vi "Uruchomienie_old.vi"() -> ()   [LabVIEW 2015]
uses:
  Typedefs/Analiza.ctl
  Typedefs/dane.ctl
  Typedefs/mqttinputs.ctl
  Libraries/MQTT.lvlibp
panel:
  in  "BtnStopPWM":bool
  out "Praca":bool
  out "DKG":bool
  in  "Cisnienie 2":T1 {"P" format="%#.1f"}
  in  "SKSVdial":T2 {"SV" format="%#.1f"; "SK" format="%#.1f"}
  in  "Start":bool
  out "Zapisane":bool
  in  "Do Bazy":bool
  out "Opis":string
  out "Tacho":dbl format="%#.0f"
  out "Moc Zamowiona":dbl
  out "Typ Palnika":string
  out "Typ Wymiennika":string
  out "SNW":string
  out "SNP":string
  out "cisnienieOK":bool
  in  "Cisnienie":bool
  in  "Analiza":T3 {"I" format="%#.0f"; "CO2" format="%#.1f"; "CO" format="%#.0f"; "O2" format="%#.1f"}
  out "SKSVOK":bool
  in  "SKSV":bool
  out "AnalizaMinKlientOK":bool
  out "AnalizaMaxKlientOK":bool
  out "AnalizaMinOK":bool
  out "AnalizaMaxOK":bool
  in  "AnalizaMinKlient":bool
  in  "AnalizaMaxKlient":bool
  in  "AnalizaMin":bool
  in  "AnalizaMax":bool
  in  "BtnMaxLufa":bool
  in  "BtnMin":bool
  in  "PWMMin":dbl=15.0
  in  "BtnMax Klient":bool
  in  "PWM Max Klient":dbl=90.0
  in  "Kas":bool
  out "Awaria":bool
  out "PWM":dbl
  in  "BtnMax":bool
  in  "PWM Max":dbl=100.0
  in  "BtnMin Klient":bool
  in  "PWMMinKlient":dbl=15.0
  in  "BtnStart":bool
  out "MOC":dbl format="%#_1g"
  in  "Uruchamia:":u16(ring) items=["------", "KAMIŃSKI JAKUB", "RADZIWON TOMASZ", "RADZIWON JAKUB", "RADZIWON MICHAŁ", "HARBANOWICZ FRANCISZEK", "JANUSZKIEWICZ JAKUB", "PIOTROWSKI DAMIAN", "WISZNIEWSKI JERZY", "BOHM ŁUKASZ", "KARPIŃSKI GRZEGORZ", "KAMIŃSKI JAKUB"]
  in  "Temat":u16(ring) items=["------"]
  in  "PWMStart":dbl=25.0
  in  "Nawiew_f":dbl=7.0
  in  "Nawiew":bool
  out "GAZ":bool
  in  "Zaplon":bool
  # "Hz"
  # "kW"
  # "21-24: 25%\npozostale 45%"
  # "%"
  # "%"
  # "Hz"
  # "%"
  # "%"
  # "%"
  # "%"
  # "Pa"
  # "mm"
  # "mm"
  # "Pmax 4%-5%\nPmin 3%-6.5%"
  # "%"
  # "%"
  # "ppm"
  # "<100ppm"
  # "uA"
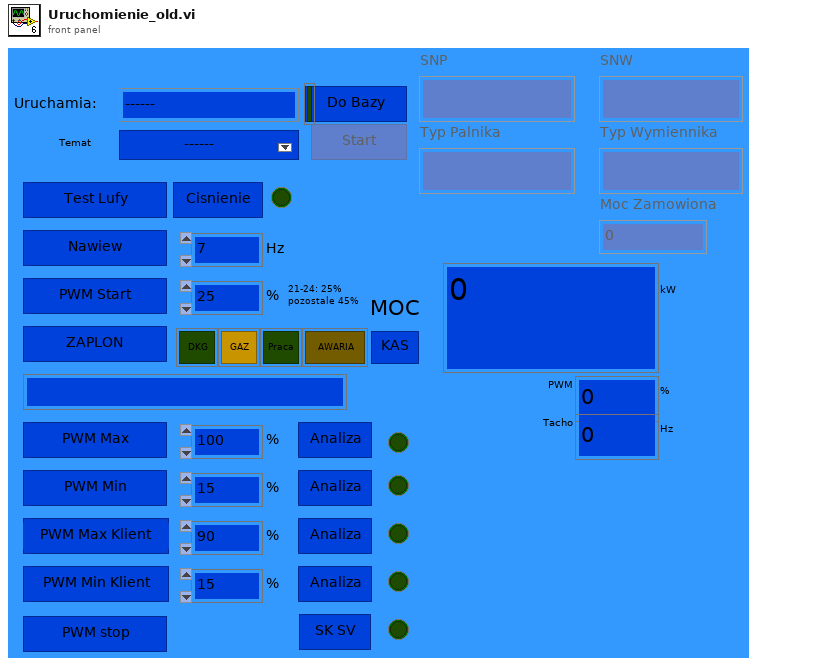
[diagram p1: front panel]
types:
  T1 = cluster{"P":dbl, "OK Button":bool, "Cancel Button":bool}
  T2 = cluster{"SK":dbl, "OK Button":bool, "Cancel Button":bool, "SV":dbl}
  T3 = typedef "Analiza.ctl" = cluster{"O2":dbl, "CO":dbl, "OK Button":bool, "Cancel Button":bool, "CO2":dbl, "I":dbl}
  T4 = typedef "MQTT.lvlibp/Broadcast Events--cluster.ctl" = cluster{"Module Did Init":refnum<user-event>, "Status Updated":refnum<user-event>, "Error Reported":refnum<user-event>, "Module Did Stop":refnum<user-event>, "Update Module Execution Status":refnum<user-event>, "Message":refnum<user-event>}
  T5 = enum8{"Enabled", "Disabled", "Disabled and Grayed Out"}
  T6 = enum32{"invalid app kind", "Development System", "Run Time System", "Student Edition", "Embedded LabVIEW", "Evaluation", "Custom"}
  T7 = typedef "dane.ctl" = cluster{"P":cluster{"max":dbl, "min":dbl, "klientmax":dbl, "klientmin":dbl}, "CO":cluster{"max":dbl, "min":dbl, "klientmax":dbl, "klientmin":dbl}, "CO2":cluster{"max":dbl, "min":dbl, "klientmax":dbl, "klientmin":dbl}, "O2":cluster{"max":dbl, "min":dbl, "klientmax":dbl, "klientmin":dbl}, "I":cluster{"max":dbl, "min":dbl, "klientmax":dbl, "klientmin":dbl}, "n":cluster{"max":dbl, "min":dbl, "klientmax":dbl, "klientmin":dbl}, "pwm":cluster{"klientmax":dbl, "klientmin":dbl}, "valve":cluster{"SK":dbl, "SV":dbl}, "pLufa100":dbl, "data":cluster{"Uruchomil":dbl, "Temat":string, "Podtemat":string, "Uwagi":string}}
  T8 = enum32{"Invalid", "Standard", "Closed", "Hidden", "Minimized", "Maximized"}
  T9 = typedef "mqttinputs.ctl" = cluster{"Power":dbl, "PWM":i32, "Tacho":i32, "Gaz":bool, "Awaria":bool, "dP":dbl, "Praca":bool, "DKG":bool}
  T10 = cluster{refnum<vi>[], "Core":cluster{"Current VI Reference":refnum<vi>, "Close Panel on Exit?":bool}, "controls":refnum<vi>[], "Kto-Lista":string[], "Kto-Lista-Num":i32[], "Kto":u8, "Tematy-Lista":string[], "TematyDane":string[][], "Temat":string, "Data":T7, "PWM":cluster{" start":i32, "min":i32, "max":i32, "moc":i32, "min klient":i32, "max klient":i32}, "CurrentPWM":i32, "broadcasts":variant, "Subscriptions":variant, "Inputs":T9, "Analiza":string}
  T11 = cluster{" start":i32, "min":i32, "max":i32, "moc":i32, "min klient":i32, "max klient":i32}
  T12 = cluster{"Current VI Reference":refnum<vi>, "Close Panel on Exit?":bool}
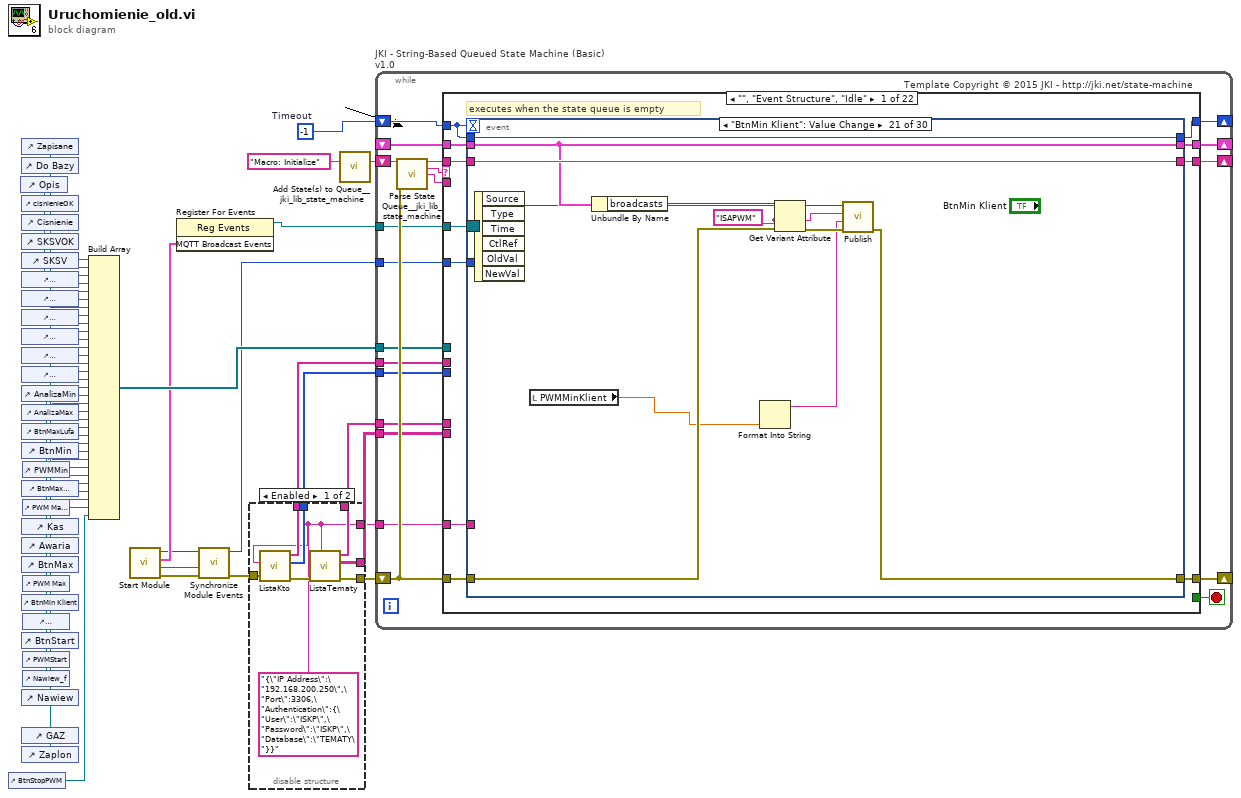
[diagram p0: block diagram]
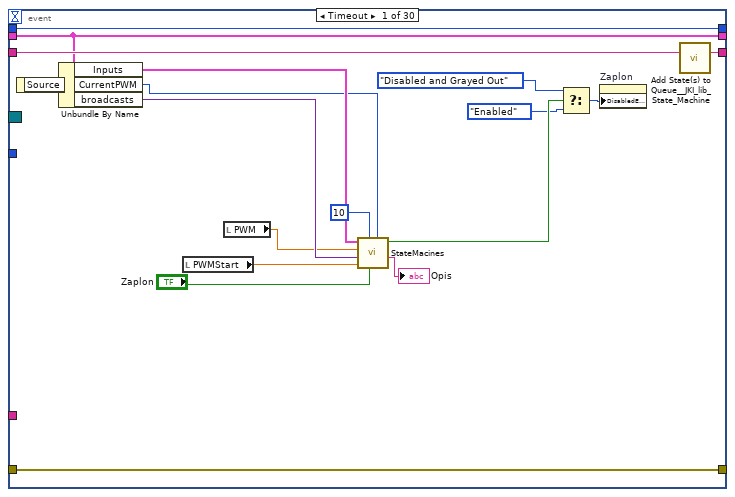
[diagram p3: hidden frame]
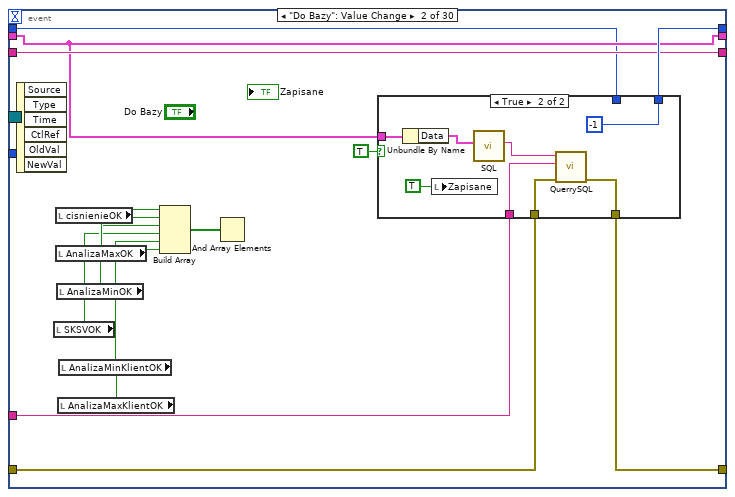
[diagram p4: hidden frame]
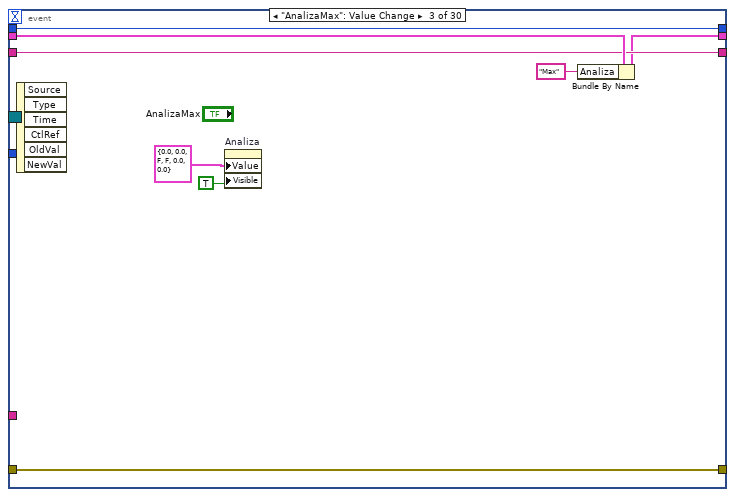
[diagram p6: hidden frame]
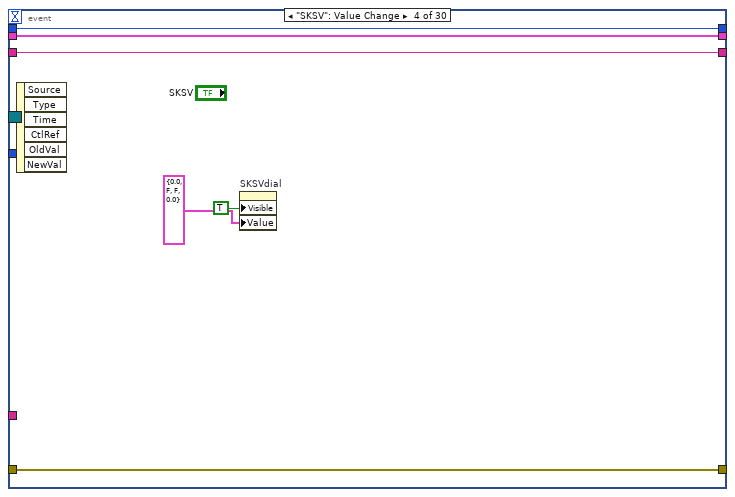
[diagram p7: hidden frame]
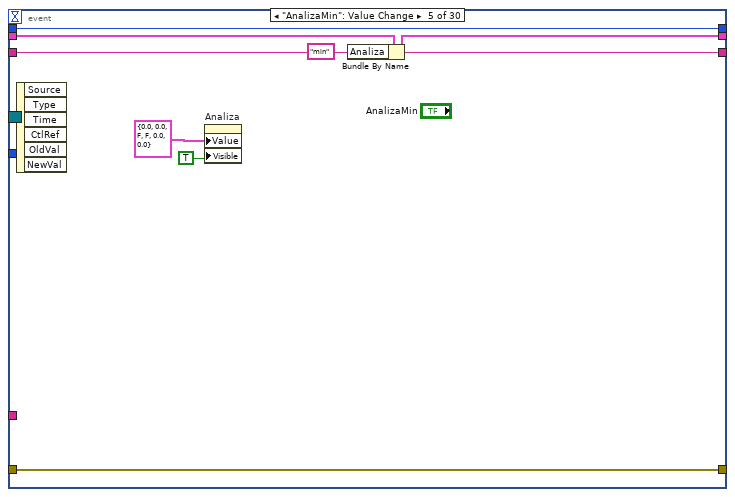
[diagram p8: hidden frame]
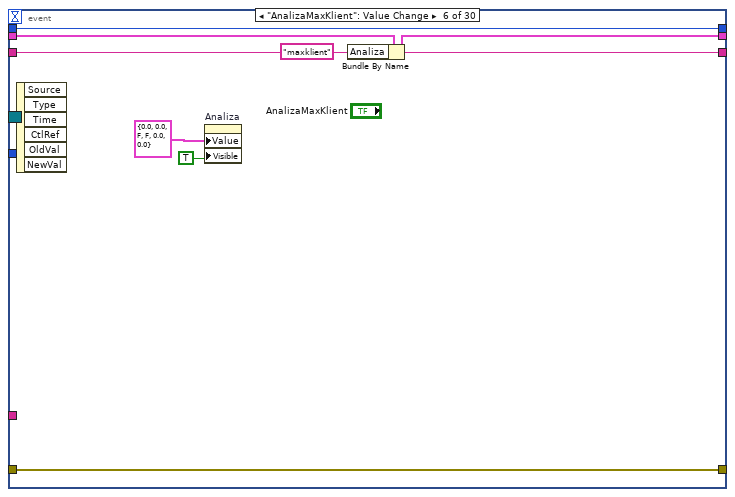
[diagram p9: hidden frame]
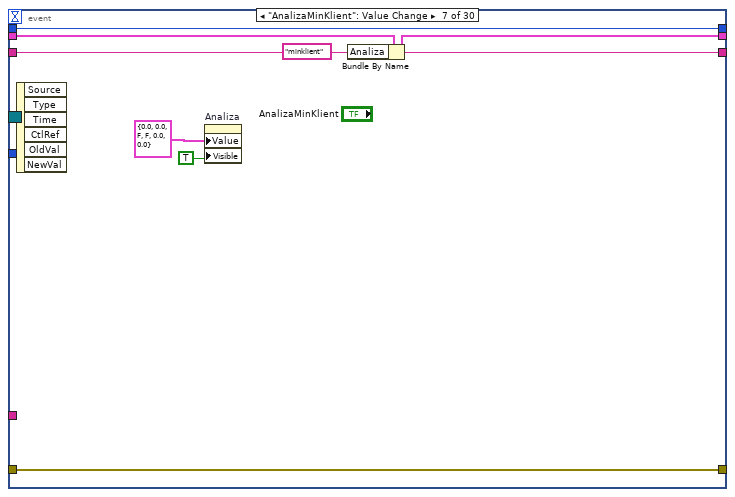
[diagram p10: hidden frame]
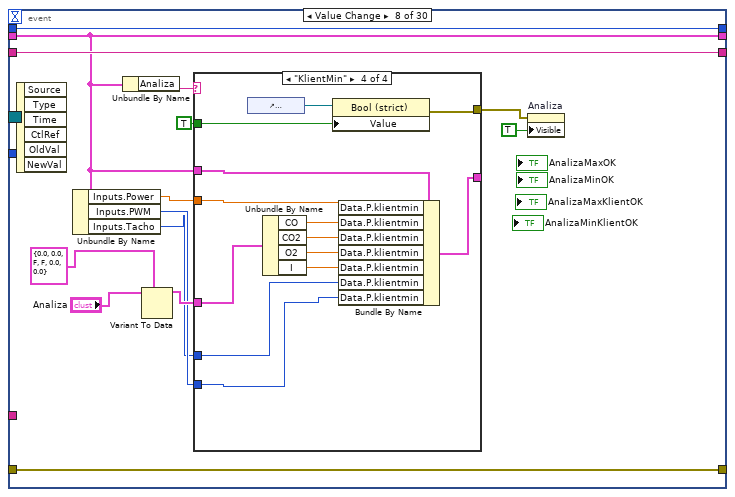
[diagram p11: hidden frame]
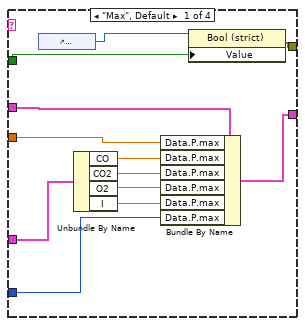
[diagram p12: hidden frame]
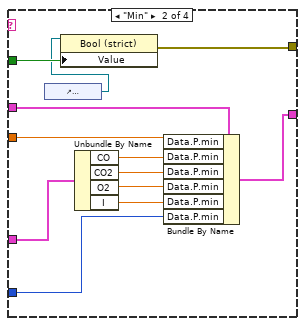
[diagram p13: hidden frame]
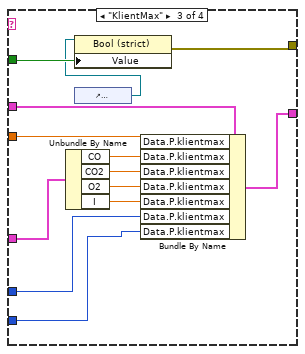
[diagram p14: hidden frame]
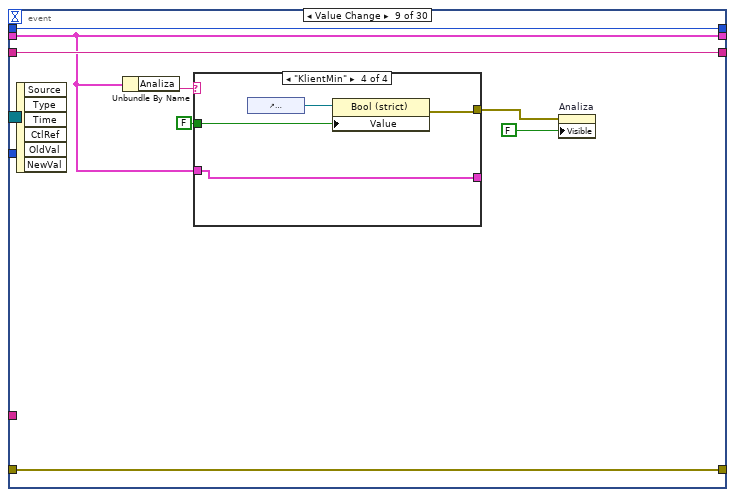
[diagram p15: hidden frame]
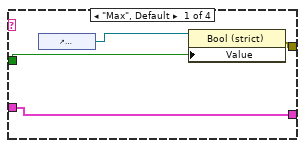
[diagram p16: hidden frame]
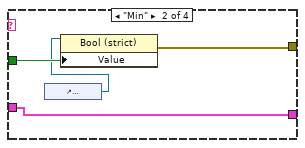
[diagram p17: hidden frame]
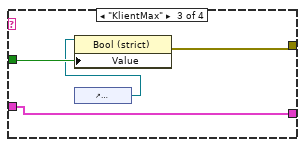
[diagram p18: hidden frame]
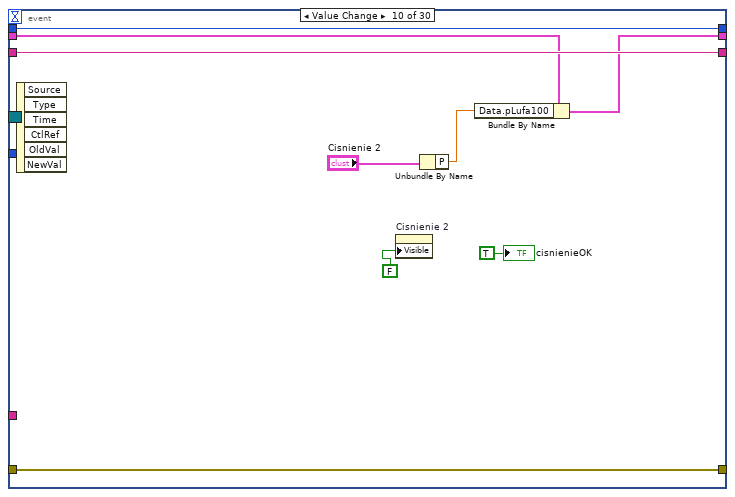
[diagram p19: hidden frame]
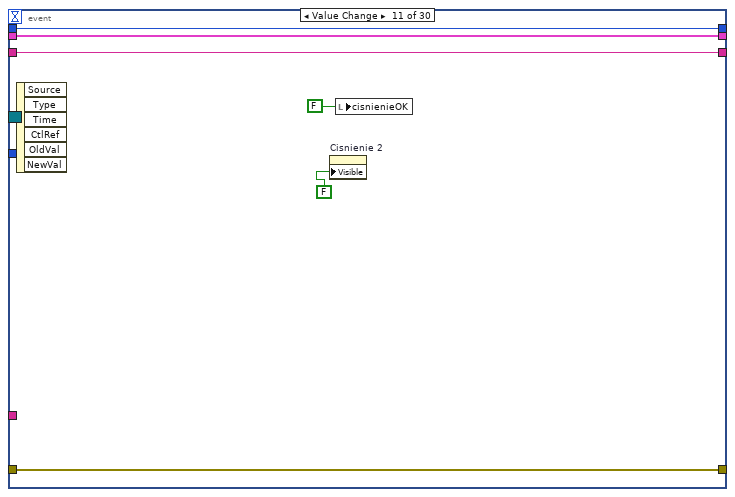
[diagram p20: hidden frame]
diagram:
  w3 = -1  # Timeout
  n1 = control-ref of="BtnStopPWM"() -> (w1:refnum<vi>)
  n2 = control-ref of="Opis"() -> (w48:refnum<vi>)
  n3 = control-ref of="Zapisane"() -> (w50:refnum<vi>)
  n4 = control-ref of="Do Bazy"() -> (w49:refnum<vi>)
  n5 = control-ref of="cisnienieOK"() -> (w47:refnum<vi>)
  n6 = control-ref of="Cisnienie"() -> (w46:refnum<vi>)
  n7 = control-ref of="SKSVOK"() -> (w45:refnum<vi>)
  n8 = control-ref of="SKSV"() -> (w44:refnum<vi>)
  n9 = control-ref of="AnalizaMinKlientOK"() -> (w43:refnum<vi>)
  n10 = control-ref of="AnalizaMaxKlientOK"() -> (w42:refnum<vi>)
  n11 = control-ref of="AnalizaMinOK"() -> (w41:refnum<vi>)
  n12 = control-ref of="AnalizaMaxOK"() -> (w40:refnum<vi>)
  n13 = control-ref of="AnalizaMinKlient"() -> (w39:refnum<vi>)
  n14 = control-ref of="AnalizaMaxKlient"() -> (w38:refnum<vi>)
  n15 = control-ref of="AnalizaMin"() -> (w37:refnum<vi>)
  n16 = control-ref of="AnalizaMax"() -> (w36:refnum<vi>)
  n17 = control-ref of="BtnMaxLufa"() -> (w35:refnum<vi>)
  n18 = control-ref of="BtnMin"() -> (w34:refnum<vi>)
  n19 = control-ref of="BtnMax Klient"() -> (w32:refnum<vi>)
  n20 = control-ref of="Kas"() -> (w30:refnum<vi>)
  n21 = control-ref of="Awaria"() -> (w29:refnum<vi>)
  n22 = control-ref of="BtnMax"() -> (w28:refnum<vi>)
  n23 = control-ref of="BtnMin Klient"() -> (w26:refnum<vi>)
  n24 = control-ref of="BtnStart"() -> (w24:refnum<vi>)
  n25 = control-ref of="Nawiew"() -> (w21:refnum<vi>)
  n26 = control-ref of="GAZ"() -> (w20:refnum<vi>)
  n27 = control-ref of="Zaplon"() -> (w19:refnum<vi>)
  n28 = control-ref of="PWMMin"() -> (w33:refnum<vi>)
  n29 = control-ref of="PWM Max Klient"() -> (w31:refnum<vi>)
  n30 = control-ref of="PWM Max"() -> (w27:refnum<vi>)
  n31 = control-ref of="PWMMinKlient"() -> (w25:refnum<vi>)
  n32 = control-ref of="PWMStart"() -> (w23:refnum<vi>)
  n33 = control-ref of="Nawiew_f"() -> (w22:refnum<vi>)
  n34 = Build Array(w50, w49, w48, w47, w46, w45, w44, w43, w42, w41, w40, w39, w38, w37, w36, w35, w34, w33, w32, w31, w30, w29, w28, w27, w26, w25, w24, w23, w22, w21, w20, w19, w1) -> (w11:refnum<vi>[])
  n35 = call "Start Module.vi"() -> ("error out"=w6:errorcluster, "Wait for Event Sync?"=w7:bool, "MQTT Broadcast Events"=w10:T4, "Module ID"=w9:i32)  [unwired: 8 in]
  n36 = register-events(w10) -> (reference out=w4:refnum<event-registration>)  [unwired: 2 in, 1 out]
  n37 = call "Synchronize Module Events.vi"("error in (no error)"=w6, "Wait for Event Sync?"=w7, "Module ID"=w9) -> ("error out"=w5:errorcluster, "Module ID (dup)"=w8:i32)  [unwired: 7 in]
  n38 = disable-structure shown="Enabled" {
    disable-tunnel: [w58 w59] -> w16
    disable-tunnel: [w56 _] -> w15
    disable-tunnel: [w55 _] -> w14
    disable-tunnel: [w54 _] -> w13
    disable-tunnel: [w53 _] -> w12
    disable-tunnel: w5 -> [w52 w59]
    disable-tunnel: [w51 _] -> w2
    frame Enabled {
      w51 = "{\"IP Address\":\"192.168.200.250\",\"Port\":3306,\"Authentication\":{\"User\":\"ISKP\",\"Password\":\"ISKP\",\"Database\":\"TEMATY\"}}" ("JSON string")
      n39 = call "ListaKto.vi"("error in (no error)"=w52, "Jsonconfig"=w51) -> ("error out"=w57:errorcluster, "Array"=w55:i32[], "Array 2"=w56:string[])  [unwired: 7 in]
      n40 = call "ListaTematy.vi"("Jsonconfig"=w51, "error in (no error)"=w57) -> ("error out"=w58:errorcluster, "data"=w53:string[][], "Array"=w54:string[])  [unwired: 7 in]
    }
    frame Disabled {
    }
  }
  n41 = call <vilib>:"Add State(s) to Queue__jki_lib_state_machine.vi"("State(s) in (\"\")"="Macro: Initialize") -> ("States Out"=w18:string)  [unwired: 14 in]
  n42 = while "JKI - String-Based Queued State Machine (Basic) v1.0" {
    shift-right: [w72] -> _
    shift-left: _ -> [w71]
    shift-right: [w75] -> _
    shift-left: w16 -> [w70]
    shift-right: [w74] -> _
    shift-left: w18 -> [w76]
    tunnel: w15 -> [w69]
    tunnel: w14 -> [w68]
    tunnel: w13 -> [w67]
    tunnel: w12 -> [w66]
    tunnel: w11 -> [w65]
    tunnel: w8 -> [w64]
    tunnel: w4 -> [w63]
    shift-right: [w61] -> _
    shift-left: w3 -> [w62]
    tunnel: w2 -> [w60]
    stop <- w73 stop-if-true
    # "Template Copyright © 2015 JKI - http://jki.net/state-machine"
    n43 = call <vilib>:"Parse State Queue__jki_lib_state_machine.vi"("State Queue"=w76, "Error In (no error)"=w70) -> ("Remaining States"=w78:string, "Current State"=w79:string, "Arguments"=w77:string)  [unwired: 11 in]
    n44 = case shown="\"\", \"Event Structure\", \"Idle\"" w79 {
      selector: w79 -> [_ _ w543 _ _ _ _ _ _ _ _ _ _ _ _ _ _ _ _ _ _ _]
      tunnel: w78 -> [w90 w541 w547 w567 w574 w585 w590 w619 w626 w631 w642 w647 w654 w670 w679 w691 w718 w724 w735 w740 w745 w750]
      tunnel: w77 -> [_ _ _ _ _ _ _ _ _ _ _ _ _ w655 w674 w685 _ _ _ _ _ _]
      tunnel: w71 -> [w88 w538 w545 w558 w571 w583 w587 _ w621 w628 w636 w644 w650 w666 w677 w687 w715 w721 w732 w737 w742 w747]
      tunnel: [w87 w539 w549 w564 errorcluster {"status"=FALSE, "code"=0, "source"=""} ("error out") w576 w588 w616 w622 w629 w638 w645 w652 w668 w675 w688 w716 w722 w733 w738 w743 w748] -> w75
      tunnel: w70 -> [w86 w539 w548 w564 w570 w577 w588 w616 w623 w629 w639 w645 w652 w668 w676 w689 w716 w722 w733 w738 w743 w748]
      tunnel: [w89 w540 w546 w566 w573 w584 w589 w618 w625 w630 w641 w646 w653 w669 w678 w690 w717 w723 w734 w739 w744 w749] -> w74
      tunnel: [_ _ _ _ _ TRUE _ _ _ _ _ _ _ _ _ _ _ _ _ _ _ _] -> w73
      tunnel: [w85 w538 w545 w565 w571 w583 w587 w617 w621 w628 w635 w644 w650 w666 w677 w687 w715 w721 w732 w737 w742 w747] -> w72
      tunnel: w62 -> [w82 w537 w542 w555 w568 w575 w586 w592 w620 w627 w632 w643 w651 w656 w673 w684 w714 w719 w725 w736 w741 w746]
      tunnel: w69 -> [_ _ _ _ _ _ _ w603 _ _ _ _ _ _ _ _ _ _ _ _ _ _]
      tunnel: w68 -> [_ _ _ _ _ _ _ w602 _ _ _ _ _ _ _ _ _ _ _ _ _ _]
      tunnel: w67 -> [_ _ _ _ _ _ _ w601 _ _ _ _ _ _ _ _ _ _ _ _ _ _]
      tunnel: w66 -> [_ _ _ _ _ _ _ w600 _ _ _ _ _ _ _ _ _ _ _ _ _ _]
      tunnel: w65 -> [_ _ _ w554 _ _ _ w598 _ _ _ _ _ _ _ _ _ _ _ _ _ _]
      tunnel: w64 -> [w84 _ _ _ _ w578 _ _ _ _ w640 _ _ _ _ _ _ _ _ _ _ _]
      tunnel: w63 -> [w83 _ _ _ _ w581 _ _ _ _ _ _ _ _ _ _ _ _ _ _ _ _]
      tunnel: [w81 w537 w542 w555 w568 w575 w586 w592 w620 w627 w632 w643 w651 w656 w673 w684 w714 w719 w725 w736 w741 w746] -> w61
      tunnel: w60 -> [w80 _ _ _ _ _ _ _ _ _ _ _ _ _ _ _ _ _ _ _ _ _]
      frame "", "Event Structure", "Idle" {
        # "executes when the state queue is empty"
        n45 = event shown="[20] \"BtnMin Klient\": Value Change" {
          selector: w83 -> [_ _ _ _ _ _ _ _ _ _ _ _ _ _ _ _ _ _ _ _ _ _ _ _ _ _ _ _ _ _]
          dyn-events: _ -> [_ _ _ _ _ _ _ _ _ _ _ _ _ _ _ _ _ _ _ _ _ _ _ _ _ _ _ _ _ _]
          timeout: w82 -> [_ _ _ _ _ _ _ _ _ _ _ _ _ _ _ _ _ _ _ _ _ _ _ _ _ _ _ _ _ _]
          tunnel: w90 -> [w107 w121 w137 w146 w154 w162 w170 w184 w242 w267 w273 w283 w289 w295 w315 w329 w338 w363 w375 w386 w398 w410 w422 w434 w454 w464 w498 w504 w526 w536]
          tunnel: [w106 w121 w137 w146 w154 w162 w170 w184 w242 w267 w273 w283 w289 w295 w315 w329 w338 w363 w375 w386 w398 w410 w422 w434 w454 w464 w498 w505 w526 w535] -> w89
          tunnel: w88 -> [w100 w120 w138 w144 w152 w160 w168 w174 w237 w263 w271 w277 w287 w293 w313 w327 w336 w361 w373 w384 w396 w408 w420 w432 w452 w457 w496 w506 w524 w533]
          tunnel: [w105 w117 w139 w145 w153 w161 w169 w183 w241 w266 w272 w282 w288 w294 w301 w321 w333 w358 w370 w381 w393 w405 w417 w429 w436 w459 w494 w502 w509 w534] -> w87
          tunnel: w86 -> [w105 w118 w139 w145 w153 w161 w169 w183 w241 w266 w272 w282 w288 w294 w302 w320 w332 w357 w369 w380 w392 w404 w416 w428 w447 w459 w494 w502 w509 w534]
          tunnel: [w100 w120 w136 w144 w148 w156 w164 w174 w237 w262 w271 w276 w287 w293 w313 w327 w336 w361 w373 w384 w396 w408 w420 w432 w452 w456 w495 w506 w525 w533] -> w85
          tunnel: w84 -> [_ _ _ _ _ _ _ _ _ _ _ _ _ _ w305 w323 w334 w359 w371 w382 w394 w406 w418 w430 w438 _ _ _ _ _]
          tunnel: w82 -> [w97 w108 w140 w143 w151 w159 w167 w182 w240 w265 w270 w281 w286 w292 w314 w328 w337 w362 w374 w385 w397 w409 w421 w433 w453 w455 w493 _ w507 w530]
          tunnel: [w97 w122 w140 w143 w151 w159 w167 w182 w240 w265 w270 w281 w286 w292 w314 w328 w337 w362 w374 w385 w397 w409 w421 w433 w453 w455 w493 500 ("Timeout") w507 w530] -> w81
          tunnel: w80 -> [_ w119 _ _ _ _ _ _ _ _ _ _ _ _ _ _ _ _ _ _ _ _ _ _ _ _ _ _ _ _]
          event Timeout {
            n46 = event-data() -> ()  [unwired: 1 in, 1 out]
            n47 = Unbundle By Name(w100) -> ("Inputs"=w99:T9, "CurrentPWM"=w91:i32, "broadcasts"=w98:variant)
            n48 = local read "PWMStart"() -> (w96:dbl)
            n49 = local read "PWM"() -> (w93:dbl)
            n50 = call "StateMacines.vi"("PWM Demand"=w91, "Operate"="Zaplon", "Purge Time"=10, "PWMStart"=w96, "broadcasts"=w98, "CurrentPWM"=w93, "Inputs"=w99) -> ("Opis"=→"Opis":string, "DisableStartBtn"=w104:bool)  [unwired: 1 in, 2 out]
            n51 = Select(t=T5."Disabled and Grayed Out" ("Disabled"), s=w104, f=T5."Enabled" ("Disabled")) -> (s? t:f=w101:T5)
            n52 = property on="Zaplon" class="Bool (strict)"("DisabledEnum"=w101) -> ()  [unwired: 2 in, 2 out]
            n53 = call <vilib>:"Add State(s) to Queue__JKI_lib_State_Machine.vi"("State(s) in (\"\")"=w107) -> ("States Out"=w106:string)  [unwired: 14 in]
          }
          event "Do Bazy": Value Change {
            n54 = event-data() -> ()  [unwired: 1 in, 6 out]
            n55 = local read "SKSVOK"() -> (w113:bool)
            n56 = local read "cisnienieOK"() -> (w116:bool)
            n57 = local read "AnalizaMaxOK"() -> (w115:bool)
            n58 = local read "AnalizaMinOK"() -> (w114:bool)
            n59 = local read "AnalizaMaxKlientOK"() -> (w111:bool)
            n60 = local read "AnalizaMinKlientOK"() -> (w112:bool)
            n61 = Build Array(w116, w115, w114, w113, w112, w111) -> (w110:bool[])
            n62 = And Array Elements(Boolean array=w110) -> ()  [unwired: 1 out]
            n63 = case shown="True" TRUE {
              tunnel: [w123 -1 ("Timeout")] -> w122
              tunnel: w120 -> [_ w131]
              tunnel: w119 -> [_ w128]
              tunnel: w118 -> [w124 w127]
              tunnel: [w124 w126] -> w117
              tunnel: w108 -> [w123 _]
              frame False {
              }
              frame True {
                n64 = Unbundle By Name(w131) -> ("Data"=w130:T7)
                n65 = local write "Zapisane"(TRUE ("Zapisane")) -> ()
                n66 = call "SQL.vi"("Data"=w130) -> ("SQL querry"=w129:string)  [unwired: 9 in, 1 out]
                n67 = call "QuerrySQL.vi"("error in (no error)"=w127, "Jsonconfig"=w128, "String"=w129) -> ("error out"=w126:errorcluster)  [unwired: 7 in, 1 out]
              }
            }
          }
          event "AnalizaMax": Value Change {
            n68 = event-data() -> ()  [unwired: 1 in, 6 out]
            n69 = property on="Analiza" class="Clust"("Value"=T3 {"O2"=0.0, "CO"=0.0, "OK Button"=FALSE, "Cancel Button"=FALSE, "CO2"=0.0, "I"=0.0} ("Analiza"), "Visible"=TRUE) -> ()  [unwired: 2 in, 2 out]
            n70 = Bundle By Name(cluster=w138, "Analiza"="Max") -> (w136:T10)
          }
          event "SKSV": Value Change {
            n71 = event-data() -> ()  [unwired: 1 in, 6 out]
            n72 = property on="SKSVdial" class="Clust"("Visible"=TRUE, "Value"=T2 {"SK"=0.0, "OK Button"=FALSE, "Cancel Button"=FALSE, "SV"=0.0} ("SKSV")) -> ()  [unwired: 2 in, 2 out]
          }
          event "AnalizaMin": Value Change {
            n73 = event-data() -> ()  [unwired: 1 in, 6 out]
            n74 = property on="Analiza" class="Clust"("Value"=T3 {"O2"=0.0, "CO"=0.0, "OK Button"=FALSE, "Cancel Button"=FALSE, "CO2"=0.0, "I"=0.0} ("Analiza"), "Visible"=TRUE) -> ()  [unwired: 2 in, 2 out]
            n75 = Bundle By Name(cluster=w152, "Analiza"="min") -> (w148:T10)
          }
          event "AnalizaMaxKlient": Value Change {
            n76 = event-data() -> ()  [unwired: 1 in, 6 out]
            n77 = property on="Analiza" class="Clust"("Value"=T3 {"O2"=0.0, "CO"=0.0, "OK Button"=FALSE, "Cancel Button"=FALSE, "CO2"=0.0, "I"=0.0} ("Analiza"), "Visible"=TRUE) -> ()  [unwired: 2 in, 2 out]
            n78 = Bundle By Name(cluster=w160, "Analiza"="maxklient") -> (w156:T10)
          }
          event "AnalizaMinKlient": Value Change {
            n79 = event-data() -> ()  [unwired: 1 in, 6 out]
            n80 = property on="Analiza" class="Clust"("Value"=T3 {"O2"=0.0, "CO"=0.0, "OK Button"=FALSE, "Cancel Button"=FALSE, "CO2"=0.0, "I"=0.0} ("Analiza"), "Visible"=TRUE) -> ()  [unwired: 2 in, 2 out]
            n81 = Bundle By Name(cluster=w168, "Analiza"="minklient") -> (w164:T10)
          }
          event Value Change {
            n82 = event-data() -> ()  [unwired: 1 in, 6 out]
            n83 = Unbundle By Name(w174) -> ("Inputs.Power"=w173:dbl, "Inputs.PWM"=w172:i32, "Inputs.Tacho"=w171:i32)
            n84 = Unbundle By Name(w174) -> ("Analiza"=w178:string)
            n85 = Variant To Data(type=T3 {"O2"=0.0, "CO"=0.0, "OK Button"=FALSE, "Cancel Button"=FALSE, "CO2"=0.0, "I"=0.0} ("Analiza"), Variant="Analiza") -> (data=w180:T3)  [unwired: 1 in, 1 out]
            n86 = case shown="\"KlientMin\"" w178 {
              tunnel: TRUE ("AnalizaMinOK") -> [w196 w208 w221 w234]
              tunnel: [w195 w207 w220 w233] -> w177
              tunnel: [w190 w202 w218 w227] -> _
              tunnel: w174 -> [w189 w201 w219 w228]
              tunnel: w180 -> [w188 w199 w217 w225]
              tunnel: w173 -> [w187 w200 w212 w226]
              tunnel: w171 -> [w186 w198 w211 w224]
              tunnel: w172 -> [_ _ w210 w223]
              frame "Max", Default {
                n87 = control-ref of="AnalizaMaxOK"() -> (w185:refnum<vi>)
                n88 = Unbundle By Name(w188) -> ("CO"=w194:dbl, "CO2"=w193:dbl, "O2"=w192:dbl, "I"=w191:dbl)
                n89 = Bundle By Name(cluster=w189, "Data.P.max"=w187, "Data.P.max"=w194, "Data.P.max"=w193, "Data.P.max"=w192, "Data.P.max"=w191, "Data.P.max"=w186) -> (w190:T10)
                n90 = property on="Property Node" class="Bool (strict)"(reference=w185, "Value"=w196) -> (error out=w195:errorcluster)  [unwired: 1 in, 1 out]
              }
              frame "Min" {
                n91 = control-ref of="AnalizaMinOK"() -> (w197:refnum<vi>)
                n92 = property on="Property Node" class="Bool (strict)"(reference=w197, "Value"=w208) -> (error out=w207:errorcluster)  [unwired: 1 in, 1 out]
                n93 = Unbundle By Name(w199) -> ("CO"=w206:dbl, "CO2"=w205:dbl, "O2"=w204:dbl, "I"=w203:dbl)
                n94 = Bundle By Name(cluster=w201, "Data.P.min"=w200, "Data.P.min"=w206, "Data.P.min"=w205, "Data.P.min"=w204, "Data.P.min"=w203, "Data.P.min"=w198) -> (w202:T10)
              }
              frame "KlientMax" {
                n95 = Unbundle By Name(w217) -> ("CO"=w213:dbl, "CO2"=w214:dbl, "O2"=w215:dbl, "I"=w216:dbl)
                n96 = control-ref of="AnalizaMaxKlientOK"() -> (w209:refnum<vi>)
                n97 = property on="Property Node" class="Bool (strict)"(reference=w209, "Value"=w221) -> (error out=w220:errorcluster)  [unwired: 1 in, 1 out]
                n98 = Bundle By Name(cluster=w219, "Data.P.klientmax"=w212, "Data.P.klientmax"=w213, "Data.P.klientmax"=w214, "Data.P.klientmax"=w215, "Data.P.klientmax"=w216, "Data.P.klientmax"=w211, "Data.P.klientmax"=w210) -> (w218:T10)
              }
              frame "KlientMin" {
                n99 = control-ref of="AnalizaMinKlientOK"() -> (w222:refnum<vi>)
                n100 = Unbundle By Name(w225) -> ("CO"=w232:dbl, "CO2"=w231:dbl, "O2"=w230:dbl, "I"=w229:dbl)
                n101 = property on="Property Node" class="Bool (strict)"(reference=w222, "Value"=w234) -> (error out=w233:errorcluster)  [unwired: 1 in, 1 out]
                n102 = Bundle By Name(cluster=w228, "Data.P.klientmin"=w226, "Data.P.klientmin"=w232, "Data.P.klientmin"=w231, "Data.P.klientmin"=w230, "Data.P.klientmin"=w229, "Data.P.klientmin"=w224, "Data.P.klientmin"=w223) -> (w227:T10)
              }
            }
            n103 = property on="Analiza" class="Clust"(error in=w177, "Visible"=TRUE) -> ()  [unwired: 1 in, 2 out]
          }
          event Value Change {
            n104 = event-data() -> ()  [unwired: 1 in, 6 out]
            n105 = Unbundle By Name(w237) -> ("Analiza"=w239:string)
            n106 = case shown="\"KlientMin\"" w239 {
              tunnel: FALSE ("AnalizaMinOK") -> [w246 w250 w254 w258]
              tunnel: [w245 w249 w253 w257] -> w236
              tunnel: [w244 w248 w252 w256] -> _
              tunnel: w237 -> [w244 w248 w252 w256]
              frame "Max", Default {
                n107 = control-ref of="AnalizaMaxOK"() -> (w243:refnum<vi>)
                n108 = property on="Property Node" class="Bool (strict)"(reference=w243, "Value"=w246) -> (error out=w245:errorcluster)  [unwired: 1 in, 1 out]
              }
              frame "Min" {
                n109 = control-ref of="AnalizaMinOK"() -> (w247:refnum<vi>)
                n110 = property on="Property Node" class="Bool (strict)"(reference=w247, "Value"=w250) -> (error out=w249:errorcluster)  [unwired: 1 in, 1 out]
              }
              frame "KlientMax" {
                n111 = control-ref of="AnalizaMaxKlientOK"() -> (w251:refnum<vi>)
                n112 = property on="Property Node" class="Bool (strict)"(reference=w251, "Value"=w254) -> (error out=w253:errorcluster)  [unwired: 1 in, 1 out]
              }
              frame "KlientMin" {
                n113 = control-ref of="AnalizaMinKlientOK"() -> (w255:refnum<vi>)
                n114 = property on="Property Node" class="Bool (strict)"(reference=w255, "Value"=w258) -> (error out=w257:errorcluster)  [unwired: 1 in, 1 out]
              }
            }
            n115 = property on="Analiza" class="Clust"(error in=w236, "Visible"=FALSE) -> ()  [unwired: 1 in, 2 out]
          }
          event "Cisnienie 2.OK Button": Value Change {
            n116 = event-data() -> ()  [unwired: 1 in, 6 out]
            n117 = property on="Cisnienie 2" class="Clust"("Visible"=FALSE) -> ()  [unwired: 2 in, 2 out]
            n118 = Unbundle By Name("Cisnienie 2") -> ("P"=w264:dbl)
            n119 = Bundle By Name(cluster=w263, "Data.pLufa100"=w264) -> (w262:T10)
            "cisnienieOK" <- TRUE ("cisnienieOK")
          }
          event "Cisnienie 2.Cancel Button": Value Change {
            n120 = event-data() -> ()  [unwired: 1 in, 6 out]
            n121 = property on="Cisnienie 2" class="Clust"("Visible"=FALSE) -> ()  [unwired: 2 in, 2 out]
            n122 = local write "cisnienieOK"(FALSE ("cisnienieOK")) -> ()
          }
          event "SKSVdial.OK Button": Value Change {
            n123 = event-data() -> ()  [unwired: 1 in, 6 out]
            n124 = property on="SKSVdial" class="Clust"("Visible"=FALSE) -> ()  [unwired: 2 in, 2 out]
            n125 = Unbundle By Name("SKSVdial") -> ("SK"=w279:dbl, "SV"=w278:dbl)
            n126 = Bundle By Name(cluster=w277, "Data.valve.SK"=w279, "Data.valve.SV"=w278) -> (w276:T10)
            "SKSVOK" <- TRUE ("SKSVOK")
          }
          event "SKSVdial.Cancel Button": Value Change {
            n127 = event-data() -> ()  [unwired: 1 in, 6 out]
            n128 = property on="SKSVdial" class="Clust"("Visible"=FALSE) -> ()  [unwired: 2 in, 2 out]
            n129 = local write "SKSVOK"(FALSE ("SKSVOK")) -> ()
          }
          event "Cisnienie": Value Change {
            n130 = event-data() -> ()  [unwired: 1 in, 6 out]
            n131 = property on="Cisnienie 2" class="Clust"("Value"=T1 {"P"=0.0, "OK Button"=FALSE, "Cancel Button"=FALSE} ("Cisnienie 2"), "Visible"=TRUE) -> ()  [unwired: 2 in, 2 out]
          }
          event "Nawiew": Value Change {
            w308 = "InverterDrive"
            w311 = "InverterEngage"
            n132 = event-data() -> ()  [unwired: 1 in, 6 out]
            n133 = case shown="False" "Nawiew" {
              tunnel: [0.0 ("Nawiew_f") w317] -> w300
              frame False {
              }
              frame True {
                n134 = local read "Nawiew_f"() -> (w317:dbl)
              }
            }
            n135 = Unbundle By Name(w313) -> ("broadcasts"=w312:variant)
            n136 = Get Variant Attribute(Variant=w312, name=w311, default value (empty Variant)=w311, error in=w302) -> (duplicate Variant=w309:variant, value=w306:string, error out=w310:errorcluster)  [unwired: 1 out]
            n137 = Boolean To (0,1)(Boolean="Nawiew") -> (0, 1=w297:i16)
            n138 = Format Into String(w297) -> (resulting string=w296:string)  [unwired: 3 in, 1 out]
            n139 = Format Into String(w300) -> (resulting string=w299:string)  [unwired: 3 in, 1 out]
            n140 = Get Variant Attribute(Variant=w309, name=w308, default value (empty Variant)=w308, error in=w310) -> (value=w307:string, error out=w304:errorcluster)  [unwired: 2 out]
            n141 = call "Publish.vi"("error in (no error)"=w304, "Payload"=w299, "Topic"=w307, "Module ID"=w305) -> ("error out"=w303:errorcluster)  [unwired: 7 in]
            n142 = call "Publish.vi"("error in (no error)"=w303, "Payload"=w296, "Topic"=w306, "Module ID"=w305) -> ("error out"=w301:errorcluster)  [unwired: 7 in]
          }
          event "Nawiew_f": Value Change {
            w325 = "InverterDrive"
            n143 = event-data() -> ()  [unwired: 1 in, 6 out]
            n144 = Unbundle By Name(w327) -> ("broadcasts"=w326:variant)
            n145 = Format Into String("Nawiew_f") -> (resulting string=w319:string)  [unwired: 3 in, 1 out]
            n146 = Get Variant Attribute(Variant=w326, name=w325, default value (empty Variant)=w325, error in=w320) -> (value=w324:string, error out=w322:errorcluster)  [unwired: 2 out]
            n147 = call "Publish.vi"("error in (no error)"=w322, "Payload"=w319, "Topic"=w324, "Module ID"=w323) -> ("error out"=w321:errorcluster)  [unwired: 7 in]
          }
          event "PWM Max", "PWMMin", "PWM Max Klient", "PWMMinKlient", "PWMStart": Value Change {
            n148 = event-data() -> ("NewVal"=w331:dbl)  [unwired: 1 in, 5 out]
            n149 = Unbundle By Name(w336) -> ("Inputs.Praca"=w330:bool, "broadcasts"=w335:variant)
            n150 = case shown="False" w330 {
              tunnel: w335 -> [_ w348]
              tunnel: w334 -> [_ w345]
              tunnel: [w339 w343] -> w333
              tunnel: w332 -> [w339 w342]
              tunnel: w331 -> [_ w340]
              frame False {
              }
              frame True {
                w347 = "ISAPWM"
                n151 = Format Into String(w340) -> (resulting string=w341:string)  [unwired: 3 in, 1 out]
                n152 = Get Variant Attribute(Variant=w348, name=w347, default value (empty Variant)=w347, error in=w342) -> (value=w346:string, error out=w344:errorcluster)  [unwired: 2 out]
                n153 = call "Publish.vi"("error in (no error)"=w344, "Payload"=w341, "Topic"=w346, "Module ID"=w345) -> ("error out"=w343:errorcluster)  [unwired: 7 in]
              }
            }
          }
          event "BtnMaxLufa": Value Change {
            w356 = "ISAPWM"
            n154 = event-data() -> ()  [unwired: 1 in, 6 out]
            n155 = Unbundle By Name(w361) -> ("broadcasts"=w360:variant)
            n156 = Select(t=100, s="BtnMaxLufa", f=0) -> (s? t:f=w349:i32)
            n157 = Format Into String(w349) -> (resulting string=w353:string)  [unwired: 3 in, 1 out]
            n158 = Get Variant Attribute(Variant=w360, name=w356, default value (empty Variant)=w356, error in=w357) -> (value=w355:string, error out=w354:errorcluster)  [unwired: 2 out]
            n159 = call "Publish.vi"("error in (no error)"=w354, "Payload"=w353, "Topic"=w355, "Module ID"=w359) -> ("error out"=w358:errorcluster)  [unwired: 7 in]
          }
          event "BtnMax Klient": Value Change {
            w368 = "ISAPWM"
            n160 = event-data() -> ()  [unwired: 1 in, 6 out]
            n161 = local read "PWM Max Klient"() -> (w364:dbl)
            n162 = Unbundle By Name(w373) -> ("broadcasts"=w372:variant)
            n163 = Format Into String(w364) -> (resulting string=w365:string)  [unwired: 3 in, 1 out]
            n164 = Get Variant Attribute(Variant=w372, name=w368, default value (empty Variant)=w368, error in=w369) -> (value=w367:string, error out=w366:errorcluster)  [unwired: 2 out]
            n165 = call "Publish.vi"("error in (no error)"=w366, "Payload"=w365, "Topic"=w367, "Module ID"=w371) -> ("error out"=w370:errorcluster)  [unwired: 7 in]
          }
          event "BtnStopPWM": Value Change {
            w379 = "ISAPWM"
            n166 = event-data() -> ()  [unwired: 1 in, 6 out]
            n167 = Unbundle By Name(w384) -> ("broadcasts"=w383:variant)
            n168 = Get Variant Attribute(Variant=w383, name=w379, default value (empty Variant)=w379, error in=w380) -> (value=w378:string, error out=w377:errorcluster)  [unwired: 2 out]
            n169 = call "Publish.vi"("error in (no error)"=w377, "Payload"="0", "Topic"=w378, "Module ID"=w382) -> ("error out"=w381:errorcluster)  [unwired: 7 in]
          }
          event "BtnMin Klient": Value Change {
            w391 = "ISAPWM"
            n170 = event-data() -> ()  [unwired: 1 in, 6 out]
            n171 = local read "PWMMinKlient"() -> (w387:dbl)
            n172 = Unbundle By Name(w396) -> ("broadcasts"=w395:variant)
            n173 = Format Into String(w387) -> (resulting string=w388:string)  [unwired: 3 in, 1 out]
            n174 = Get Variant Attribute(Variant=w395, name=w391, default value (empty Variant)=w391, error in=w392) -> (value=w390:string, error out=w389:errorcluster)  [unwired: 2 out]
            n175 = call "Publish.vi"("error in (no error)"=w389, "Payload"=w388, "Topic"=w390, "Module ID"=w394) -> ("error out"=w393:errorcluster)  [unwired: 7 in]
          }
          event "BtnMax": Value Change {
            w403 = "ISAPWM"
            n176 = event-data() -> ()  [unwired: 1 in, 6 out]
            n177 = local read "PWM Max"() -> (w399:dbl)
            n178 = Unbundle By Name(w408) -> ("broadcasts"=w407:variant)
            n179 = Format Into String(w399) -> (resulting string=w400:string)  [unwired: 3 in, 1 out]
            n180 = Get Variant Attribute(Variant=w407, name=w403, default value (empty Variant)=w403, error in=w404) -> (value=w402:string, error out=w401:errorcluster)  [unwired: 2 out]
            n181 = call "Publish.vi"("error in (no error)"=w401, "Payload"=w400, "Topic"=w402, "Module ID"=w406) -> ("error out"=w405:errorcluster)  [unwired: 7 in]
          }
          event "BtnMin": Value Change {
            w415 = "ISAPWM"
            n182 = event-data() -> ()  [unwired: 1 in, 6 out]
            n183 = local read "PWMMin"() -> (w411:dbl)
            n184 = Unbundle By Name(w420) -> ("broadcasts"=w419:variant)
            n185 = Format Into String(w411) -> (resulting string=w412:string)  [unwired: 3 in, 1 out]
            n186 = Get Variant Attribute(Variant=w419, name=w415, default value (empty Variant)=w415, error in=w416) -> (value=w414:string, error out=w413:errorcluster)  [unwired: 2 out]
            n187 = call "Publish.vi"("error in (no error)"=w413, "Payload"=w412, "Topic"=w414, "Module ID"=w418) -> ("error out"=w417:errorcluster)  [unwired: 7 in]
          }
          event "BtnStart": Value Change {
            w427 = "ISAPWM"
            n188 = event-data() -> ()  [unwired: 1 in, 6 out]
            n189 = local read "PWMStart"() -> (w423:dbl)
            n190 = Unbundle By Name(w432) -> ("broadcasts"=w431:variant)
            n191 = Format Into String(w423) -> (resulting string=w424:string)  [unwired: 3 in, 1 out]
            n192 = Get Variant Attribute(Variant=w431, name=w427, default value (empty Variant)=w427, error in=w428) -> (value=w426:string, error out=w425:errorcluster)  [unwired: 2 out]
            n193 = call "Publish.vi"("error in (no error)"=w425, "Payload"=w424, "Topic"=w426, "Module ID"=w430) -> ("error out"=w429:errorcluster)  [unwired: 7 in]
          }
          event "Kas": Value Change {
            w441 = "ISAPWM"
            w450 = "ISAKASAWAR"
            n194 = event-data() -> ("NewVal"=w444:bool)  [unwired: 1 in, 5 out]
            n195 = Unbundle By Name(w452) -> ("broadcasts"=w451:variant)
            n196 = local read "PWMStart"() -> (w435:dbl)
            n197 = Boolean To (0,1)(Boolean=w444) -> (0, 1=w445:i16)
            n198 = Format Into String(w445) -> (resulting string=w446:string)  [unwired: 3 in, 1 out]
            n199 = Format Into String(w435) -> (resulting string=w437:string)  [unwired: 3 in, 1 out]
            n200 = Get Variant Attribute(Variant=w451, name=w450, default value (empty Variant)=w450, error in=w447) -> (duplicate Variant=w439:variant, value=w449:string, error out=w448:errorcluster)  [unwired: 1 out]
            n201 = call "Publish.vi"("error in (no error)"=w448, "Payload"=w446, "Topic"=w449, "Module ID"=w438) -> ("error out"=w440:errorcluster)  [unwired: 7 in]
            n202 = Get Variant Attribute(Variant=w439, name=w441, default value (empty Variant)=w441, error in=w440) -> (value=w442:string, error out=w443:errorcluster)  [unwired: 2 out]
            n203 = call "Publish.vi"("error in (no error)"=w443, "Payload"=w437, "Topic"=w442, "Module ID"=w438) -> ("error out"=w436:errorcluster)  [unwired: 7 in]
          }
          event User Event {
            n204 = event-data() -> ("Message"=w458:string, "Topic"=w462:string)  [unwired: 1 in, 4 out]
            n205 = Unbundle By Name(w457) -> ("Subscriptions"=w463:variant)
            n206 = Get Variant Attribute(Variant=w463, name=w462, default value (empty Variant)="" ("Topic"), error in=w459) -> (value=w461:string)  [unwired: 3 out]
            n207 = case shown="\"ISA010Status\"" w461 {
              tunnel: w458 -> [_ w479 w492]
              tunnel: w457 -> [w465 w477 w491]
              tunnel: [w465 w475 w490] -> w456
              frame Default {
              }
              frame "ISA010Status" {
                w483 = 77
                n208 = Unflatten From JSON(path=string[] ["PWM"], JSON string=w479, type and defaults=w483) -> (value=w472:i32, error out=w486:errorcluster)  [unwired: 4 in]
                "PWM" <- w472
                n209 = Unflatten From JSON(path=string[] ["Imp"], JSON string=w479, type and defaults=w483, error in (no error)=w486) -> (value=w471:i32, error out=w484:errorcluster)  [unwired: 3 in]
                "Tacho" <- w471
                n210 = Unflatten From JSON(path=string[] ["Inputs"], JSON string=w479, type and defaults=w483, error in (no error)=w484) -> (value=w474:i32, error out=w481:errorcluster)  [unwired: 3 in]
                n211 = Number To Boolean Array(number=w474) -> (Boolean array=w473:bool[])
                n212 = Index Array(array=w473, index #1=4 ("index")) -> (element #1=w469:bool, element #2=w468:bool, element #3=w466:bool, element #4=→"GAZ":bool)  [unwired: 3 in]
                "Awaria" <- w468
                "DKG" <- w466
                "Praca" <- w469
                n213 = Unflatten From JSON(path=string[] ["dP"], JSON string=w479, type and defaults=0.0, error in (no error)=w481) -> (value=w476:dbl)  [unwired: 3 in, 1 out]
                n214 = Bundle By Name(cluster=w477, "Inputs.PWM"=w472, "Inputs.Tacho"=w471, "Inputs.Gaz"=w466, "Inputs.Awaria"=w468, "Inputs.dP"=w476, "Inputs.Praca"=w469, "Inputs.DKG"=w466) -> (w475:T10)
              }
              frame "OmegaMoc" {
                n215 = Scan From String(format string="%.;%f", input string=w492) -> (output 1=w489:dbl)  [unwired: 3 in, 3 out]
                "MOC" <- w489
                n216 = Bundle By Name(cluster=w491, "Inputs.Power"=w489) -> (w490:T10)
              }
            }
          }
          event "Uruchamia:": Value Change {
            n217 = event-data() -> ("NewVal"=w497:u16)  [unwired: 1 in, 5 out]
            n218 = Unbundle By Name(w496) -> ("Kto-Lista-Num"=w500:i32[])
            n219 = Index Array(array=w500, index=w497) -> (element=w499:i32)
            n220 = Bundle By Name(cluster=w496, "Kto"=w499, "Data.data.Uruchomil"=w499) -> (w495:T10)
          }
          event "Start": Value Change {
            n221 = event-data() -> ()  [unwired: 1 in, 6 out]
            n222 = call <vilib>:"Add State(s) to Queue__JKI_lib_State_Machine.vi"("State(s) in Front (\"\")"="UI: Controls >> ON" ("State(s) at Back (\"\")"), "State(s) in (\"\")"=w504) -> ("States Out"=w505:string)  [unwired: 13 in]
          }
          event "Temat": Value Change {
            n223 = event-data() -> ("NewVal"=w529:u16)  [unwired: 1 in, 5 out]
            n224 = Unbundle By Name(w524) -> ("Tematy-Lista"=w528:string[], "TematyDane"=w527:string[][])
            n225 = call "TematyDane.vi"("Value"=w529, "TematyDane in"=w527, "Tematy-Lista"=w528) -> ("Array"=w521:i32[], "Dane"=w520:string[], "Podtemat"=w523:string, "Temat"=w522:string)  [unwired: 5 in]
            n226 = Index Array(array=w520) -> (element #1=→"SNW":string, element #2=→"SNP":string, element #3=→"Typ Wymiennika":string, element #4=→"Typ Palnika":string)  [unwired: 4 in]
            n227 = Index Array(array=w521) -> (element #1=w515:i32, element #2=w514:i32, element #3=w513:i32, element #4=w512:i32, element #5=w511:i32, element #6=w510:i32)  [unwired: 6 in]
            "Moc Zamowiona" <- w512
            n228 = local write "Zapisane"(FALSE ("Zapisane")) -> ()
            n229 = local write "PWMStart"(w515) -> ()
            n230 = Bundle By Name(cluster=w524, "Temat"=w522, "Data.data.Temat"=w522, "Data.data.Podtemat"=w523, "PWM.start"=w515, "PWM.min"=w514, "PWM.max"=w513, "PWM.moc"=w512, "PWM.min klient"=w511, "PWM.max klient"=w510) -> (w525:T10)
            n231 = local write "PWM Max"(w513) -> ()
            n232 = local write "PWMMin"(w514) -> ()
            n233 = local write "PWM Max Klient"(w511) -> ()
            n234 = local write "PWMMinKlient"(w510) -> ()
          }
          event Panel Close? {
            # "Discard the event because we'll close the front panel ourselves in Macro: Exit"
            # "Close Panel button (pressed) Event\n(this executes Macro: Exit to terminate the VI)"
            n235 = event-data() -> ()  [unwired: 1 in, 1 out]
            n236 = event-data("Discard?"=TRUE) -> ()  [unwired: 1 in, 1 out]
            n237 = call <vilib>:"Add State(s) to Queue__JKI_lib_State_Machine.vi"("State(s) in Front (\"\")"="Macro: Exit", "State(s) in (\"\")"=w536) -> ("States Out"=w535:string)  [unwired: 13 in]
          }
        }
      }
      frame "---------- Core ----------" {
        # "Do not put any code in this frame.\n(it is a separator no-op)"
        n238 = call <vilib>:"Add State(s) to Queue__JKI_lib_State_Machine.vi"("State(s) in (\"\")"=w541) -> ("States Out"=w540:string)  [unwired: 14 in]
      }
      frame Default {
        w552 = 42 items=["No error", "Argument error", "Memory is full", "Out of zone", "End of file", "File already open", "Generic file I/O error", "File not found", "File permission error", "Disk is full", "Duplicate path", "Too many files open", "System feature not enabled", "Resource file not found", "Cannot add resource", "Resource not found", "Image not found", "Image memory error", "Pen does not exist", "Config type invalid", "Config token not found", "Config parse error", "Config memory error", "Bad external code format", "Bad external code offset", "External code not present", "Null window", "Destroy window error", "Null menu", "Print aborted", "Bad print record", "Print driver error", "Windows error during printing", "Memory error during printing", "Print dialog error", "Generic print error", "Invalid device refnum", "Device not found", "Device parameter error", "Device unit error", "Cannot open device", "Device call aborted", "Generic error", "Cancelled by user", "Object ID too low", "Object ID too high", "Object not in heap", "Unknown heap", "Unknown object (invalid DefProc)", "Unknown object (DefProc not in table)", "Message out of range", "Invalid (null) method", "Unknown message", "Manager call not supported", "Bad address", "Network operation in progress", "Network operation timed out", "Connection is busy", "Network attribute not supported", "Network error", "Address in use", "System out of memory", "Connection aborted", "Connection refused", "Not connected", "Already connected", "Connection closed", "Initialization error (interapplication manager)", "Bad occurrence", "Wait on unbound occurrence handler", "Occurrence queue overflow", "Datalog type conflict", "Unused", "Unrecognized type (interapplication manager)", "Memory corrupt", "Failed to make temporary DLL", "Old CIN version", "Drag socket not found", "Failed to load drop-object", "Failed to register OLE object", "Failed to release OLE object", "Format specifier type mismatch", "Unknown format specifier", "Too few format specifiers", "Too many format specifiers", "Scan failed", "Newer CIN version", "Error converting to variant", "Runtime menu error", "Password tampered", "Variant attribute not found", "Incompatible variant data type", "Event data is not available", "Event Store is not present", "Occurrence is not found", "Event Queue is not created", "Event info is not available", "Refnum passed is NULL", "Error retrieving Class GUID", "Error retrieving CoClass GUID", "Error retrieving TypeLib GUID.", "Bad built application magic bytes.", "Specific driver is different from the specific driver associated with the Logical Name.", "There is no session opened to the class driver.", "Max Error", "MAX - Error with config objects", "MAX - Error loading configuration", "MAX - Group not supported"]
        # "Current State"
        # "Do not delete, rename, or modify this frame.\n(this is used to capture unhandled states and typos)"
        # "Handle mistyped state name (developer tool)"
        n239 = Format Into String(format string="Software Exception: Unhandled State \"%s\"." ("message"), error in=w548, w543) -> (resulting string=w551:string, error out=w550:errorcluster)  [unwired: 1 in]
        n240 = call <vilib>:"Error Cluster From Error Code.vi"("show call chain? (False)"=TRUE, "error in (no error)"=w550, "error message (\"\")"=w551, "error code (0)"=w552) -> ("error out"=w549:errorcluster)  [unwired: 5 in]
        n241 = call <vilib>:"Add State(s) to Queue__JKI_lib_State_Machine.vi"("State(s) in (\"\")"=w547) -> ("States Out"=w546:string)  [unwired: 14 in]
      }
      frame "Initialize Core Data" {
        # "Do not delete, rename, or modify this frame.\n(this is used to determine panel behavior on exit)"
        # "originally closed?"
        # "exe?"
        # "If panel starts closed or is an EXE, then close it when we exit"
        n242 = property class="VI"() -> ("Front Panel.Open"=w563:bool)  [unwired: 2 in, 2 out]
        n243 = property class="App"() -> ("App.Kind"=w562:T6)  [unwired: 2 in, 2 out]
        n244 = control-ref of="Current VI Reference"() -> (w556:refnum<vi>)
        n245 = Not(x=w563) -> (.not. x?=w560:bool)
        n246 = Equal?(x=w562, y=T6."Run Time System" ("Application:Kind")) -> (x = y?=w559:bool)
        n247 = Or(x=w560, y=w559) -> (x .or. y?=w557:bool)
        n248 = Bundle By Name(cluster=w558, "Core.Current VI Reference"=w556, "Core.Close Panel on Exit?"=w557, "controls"=w554) -> (w565:T10)
        n249 = call <vilib>:"Add State(s) to Queue__JKI_lib_State_Machine.vi"("State(s) in (\"\")"=w567) -> ("States Out"=w566:string)  [unwired: 14 in]
      }
      frame "Error Handler" {
        # "Unhandled Error -- Display it"
        # "Handle any errors here.\nYou can also output any states to clean-up after errors occur"
        # "Clear error"
        n250 = call <vilib>:"General Error Handler.vi"("error in (no error)"=w570) -> ()  [unwired: 10 in, 5 out]
        n251 = call <vilib>:"Add State(s) to Queue__JKI_lib_State_Machine.vi"("State(s) in Front (\"\")"="/* Post Error States", "State(s) in (\"\")"=w574) -> ("States Out"=w573:string)  [unwired: 13 in]
      }
      frame "Exit" {
        # "Do not put any code in this frame.\n(No errors that occur here will be handled.)"
        n252 = Unregister For Events(event registration refnum=w581, error in=w577) -> (error out=w579:errorcluster)
        n253 = call "disconnect.vi"("error in (no error)"=w579, "Module ID"=w578) -> ("error out"=w580:errorcluster)  [unwired: 9 in]
        n254 = call "Stop Module.vi"("error in (no error)"=w580, "Module ID"=w578) -> ("error out"=w576:errorcluster)  [unwired: 9 in]
        n255 = call <vilib>:"Add State(s) to Queue__JKI_lib_State_Machine.vi"("State(s) in (\"\")"=w585) -> ("States Out"=w584:string)  [unwired: 14 in]
      }
      frame "---------- Data ----------" {
        # "Do not put any code in this frame.\n(It is a separator no-op. You can make a copy of this frame to create a new Data frame)"
        n256 = call <vilib>:"Add State(s) to Queue__JKI_lib_State_Machine.vi"("State(s) in (\"\")"=w590) -> ("States Out"=w589:string)  [unwired: 14 in]
      }
      frame "Data: Initialize" {
        w591 = ""  # Analiza
        w593 = T9 {"Power"=0.0, "PWM"=0, "Tacho"=0, "Gaz"=FALSE, "Awaria"=FALSE, "dP"=0.0, "Praca"=FALSE, "DKG"=FALSE}  # Inputs
        w594 = variant  # Subscriptions
        w595 = variant  # broadcasts
        w596 = 0  # CurrentPWM
        w597 = T11 {" start"=45, "min"=10, "max"=100, "moc"=100, "min klient"=10, "max klient"=100}  # PWM
        w607 = string[][] []  # TematyDane
        w604 = ""  # Temat
        w608 = string[] []  # Tematy-Lista
        w613 = i32[] []  # Kto-Lista-Num
        w609 = u8 0  # Kto
        w612 = string[] []  # Kto-Lista
        w614 = refnum<vi>[] []  # controls
        w615 = T12 {"Current VI Reference"=refnum, "Close Panel on Exit?"=FALSE}  # Core
        # "Data names and types of shift register data are defined by this bundle."
        # "Initialize the shift-register data, here.\n(data names are defined by what you wire into the bundle function)"
        n257 = Insert Into Array(array=w612, new element=w603) -> (w611:string[])  [unwired: 1 in]
        n258 = Insert Into Array(array=w613, new element=w602) -> (w610:i32[])  [unwired: 1 in]
        n259 = Insert Into Array(array=w607, new element=w600) -> (w605:string[][])  [unwired: 2 in]
        n260 = Insert Into Array(array=w608, new element=w601) -> (w606:string[])  [unwired: 1 in]
        n261 = Bundle(w598, "Core"=w615, "controls"=w614, "Kto-Lista"=w611, "Kto-Lista-Num"=w610, "Kto"=w609, "Tematy-Lista"=w606, "TematyDane"=w605, "Temat"=w604, "Data"=T7 {"P"={"max"=0.0, "min"=0.0, "klientmax"=0.0, "klientmin"=0.0}, "CO"={"max"=0.0, "min"=0.0, "klientmax"=0.0, "klientmin"=0.0}, "CO2"={"max"=0.0, "min"=0.0, "klientmax"=0.0, "klientmin"=0.0}, "O2"={"max"=0.0, "min"=0.0, "klientmax"=0.0, "klientmin"=0.0}, "I"={"max"=0.0, "min"=0.0, "klientmax"=0.0, "klientmin"=0.0}, "n"={"max"=0.0, "min"=0.0, "klientmax"=0.0, "klientmin"=0.0}, "pwm"={"klientmax"=0.0, "klientmin"=0.0}, "valve"={"SK"=0.0, "SV"=0.0}, "pLufa100"=0.0, "data"={"Uruchomil"=0.0, "Temat"="", "Podtemat"="", "Uwagi"=""}}, "PWM"=w597, "CurrentPWM"=w596, "broadcasts"=w595, "Subscriptions"=w594, "Inputs"=w593, "Analiza"=w591) -> (w617:T10)  [unwired: 1 in]
        n262 = call <vilib>:"Add State(s) to Queue__JKI_lib_State_Machine.vi"("State(s) in (\"\")"=w619) -> ("States Out"=w618:string)  [unwired: 14 in]
      }
      frame "Data: Cleanup" {
        # "Cleanup any data and references, here.\n(this is called automatically, by the Macro: Exit)"
        n263 = Unbundle By Name(w621) -> ("Core.Current VI Reference"=w624:refnum<vi>)
        n264 = Close Reference(reference=w624, error in (no error)=w623) -> (error out=w622:errorcluster)
        n265 = call <vilib>:"Add State(s) to Queue__JKI_lib_State_Machine.vi"("State(s) in (\"\")"=w626) -> ("States Out"=w625:string)  [unwired: 14 in]
      }
      frame "------MQTT--------" {
        # "Do not put any code in this frame.\n(It is a separator no-op. You can make a copy of this frame to create a new Data frame)"
        n266 = call <vilib>:"Add State(s) to Queue__JKI_lib_State_Machine.vi"("State(s) in (\"\")"=w631) -> ("States Out"=w630:string)  [unwired: 14 in]
      }
      frame "MQTT: Configure" {
        # "Do not put any code in this frame.\n(It is a separator no-op. You can make a copy of this frame to create a new Data frame)"
        n267 = call <vilib>:"Application Directory.vi"() -> ("Application Directory"=w637:path)
        n268 = call "ConfigureMQTT.vi"("error in (no error)"=w639, "base path"=w637, "Module ID"=w640) -> ("error out"=w638:errorcluster, "Subscriptions"=w633:variant, "broadcasts"=w634:variant)  [unwired: 6 in]
        n269 = Bundle By Name(cluster=w636, "broadcasts"=w634, "Subscriptions"=w633) -> (w635:T10)
        n270 = call <vilib>:"Add State(s) to Queue__JKI_lib_State_Machine.vi"("State(s) in (\"\")"=w642) -> ("States Out"=w641:string)  [unwired: 14 in]
      }
      frame "---------- UI ----------" {
        # "Do not put any code in this frame.\n(It is a separator no-op. You can make a copy of this frame to create a new UI frame)"
        n271 = call <vilib>:"Add State(s) to Queue__JKI_lib_State_Machine.vi"("State(s) in (\"\")"=w647) -> ("States Out"=w646:string)  [unwired: 14 in]
      }
      frame "UI: Initialize" {
        # "Initialize the User Interface, here.\n(this is called automatically, by the Macro: Init)"
        n272 = Unbundle By Name(w650) -> ("Kto-Lista"=w649:string[], "Tematy-Lista"=w648:string[])
        n273 = property on="Uruchamia:" class="Ring (strict)"("Strings []"=w649) -> ()  [unwired: 2 in, 2 out]
        n274 = property on="Temat" class="Ring (strict)"("Strings []"=w648) -> ()  [unwired: 2 in, 2 out]
        n275 = invoke class="VI" method="Default Vals.Reinit All"() -> ()  [unwired: 3 in, 3 out]
        n276 = call <vilib>:"Add State(s) to Queue__JKI_lib_State_Machine.vi"("State(s) in (\"\")"=w654) -> ("States Out"=w653:string)  [unwired: 14 in]
      }
      frame "UI: Controls" {
        # "Initialize the User Interface, here.\n(this is called automatically, by the Macro: Init)"
        n277 = Equal?(x=w655, y="ON") -> (x = y?=w658:bool)
        n278 = Not(x=w658) -> (.not. x?=w659:bool)
        n279 = Unbundle By Name(w666) -> ("controls"=w667:refnum<vi>[])
        n280 = Select(t=T5."Enabled" ("Disabled"), s=w659, f=T5."Disabled and Grayed Out" ("Disabled")) -> (s? t:f=w660:T5)
        n281 = Select(t=T5."Enabled" ("Disabled"), s=w658, f=T5."Disabled and Grayed Out" ("Disabled")) -> (s? t:f=w663:T5)
        n282 = for {
          tunnel: w667 -> [w672] mode=indexing
          tunnel: w663 -> [w671]
          n283 = property class="Ctl"(reference=w672, "DisabledEnum"=w671) -> ()  [unwired: 1 in, 2 out]
        }
        n284 = property on="Start" class="Bool"("DisabledEnum"=w660) -> ()  [unwired: 2 in, 2 out]
        n285 = call <vilib>:"Add State(s) to Queue__JKI_lib_State_Machine.vi"("State(s) in (\"\")"=w670) -> ("States Out"=w669:string)  [unwired: 14 in]
      }
      frame "UI: Cursor Set" {
        # "Argument"
        # "Set and Unset Cursor Busy.\n(Usage: \"UI: Cursor Set >> Busy|Idle\")"
        n286 = case shown="\"Idle\", Default" w674 {
          tunnel: w676 -> [w681 w683]
          tunnel: [w680 w682] -> w675
          frame "Idle", Default {
            n287 = call <vilib>:"Unset Busy.vi"("error in (no error)"=w681) -> ("error out"=w680:errorcluster)  [unwired: 10 in]
          }
          frame "Busy" {
            n288 = call <vilib>:"Set Busy.vi"("error in (no error)"=w683) -> ("error out"=w682:errorcluster)  [unwired: 9 in, 1 out]
          }
        }
        n289 = call <vilib>:"Add State(s) to Queue__JKI_lib_State_Machine.vi"("State(s) in (\"\")"=w679) -> ("States Out"=w678:string)  [unwired: 14 in]
      }
      frame "UI: Front Panel State" {
        # "Argument"
        # "Set Front Panel Open or Closed\n(Usage: \"UI: Front Panel State >> Open|Close\")"
        n290 = Unbundle By Name(w687) -> ("Core.Current VI Reference"=w686:refnum<vi>)
        n291 = case shown="\"Open\", Default" w685 {
          tunnel: w689 -> [w695 w708]
          tunnel: [w697 w709] -> w688
          tunnel: w686 -> [w696 w706]
          frame "Open", Default {
            n292 = property class="VI"(reference=w696, error in=w695) -> (reference out=w693:refnum<vi>, error out=w694:errorcluster, "Front Panel.Open"=w692:bool)
            n293 = case shown="True" w692 {
              tunnel: [w700 w703] -> w697
              tunnel: w694 -> [w699 w703]
              tunnel: w693 -> [w698 _]
              frame False {
                n294 = invoke class="VI" method="FP.Open"(reference=w698, error in=w699, "Activate"=TRUE, "State"=T8."Standard") -> (error out=w700:errorcluster)  [unwired: 1 in, 4 out]
              }
              frame True {
              }
            }
          }
          frame "Close" {
            n295 = property class="VI"(reference=w706, error in=w708) -> (reference out=w705:refnum<vi>, error out=w707:errorcluster, "Front Panel.Open"=w704:bool)
            n296 = case shown="True" w704 {
              tunnel: [w710 w713] -> w709
              tunnel: w707 -> [w710 w712]
              tunnel: w705 -> [_ w711]
              frame False {
              }
              frame True {
                n297 = invoke class="VI" method="FP.Close"(reference=w711, error in=w712) -> (error out=w713:errorcluster)  [unwired: 1 in, 2 out]
              }
            }
          }
        }
        n298 = call <vilib>:"Add State(s) to Queue__JKI_lib_State_Machine.vi"("State(s) in (\"\")"=w691) -> ("States Out"=w690:string)  [unwired: 14 in]
      }
      frame "---------- Macro ----------" {
        # "Do not put any code in this frame.\n(It is a separator no-op. You can make a copy of this frame to create a new Macro frame)"
        n299 = call <vilib>:"Add State(s) to Queue__JKI_lib_State_Machine.vi"("State(s) in (\"\")"=w718) -> ("States Out"=w717:string)  [unwired: 14 in]
      }
      frame "Macro: Initialize" {
        w720 = "Data: Initialize\nInitialize Core Data\nMQTT: Configure\nUI: Initialize\nUI: Front Panel State >> Open\nUI: Controls >> OFF"  # Data: Initialize Initialize Core Data MQTT: Configure UI: Initialize UI: Front Panel State >> Open UI: Controls >> OFF
        # "Initialization Macro\n(This is called once, when the VI starts)"
        n300 = call <vilib>:"Add State(s) to Queue__JKI_lib_State_Machine.vi"("State(s) in Front (\"\")"=w720, "State(s) in (\"\")"=w724) -> ("States Out"=w723:string)  [unwired: 13 in]
      }
      frame "Macro: Exit" {
        # "Exit Macro\n(This is called once, when the VI exits)"
        n301 = Unbundle By Name(w732) -> ("Core.Close Panel on Exit?"=w731:bool)
        n302 = Select(t="UI: Front Panel State >> Close", s=w731, f="") -> (s? t:f=w728:string)
        n303 = call <vilib>:"Add State(s) to Queue__JKI_lib_State_Machine.vi"("State(s) in (\"\")"=w728, "State(s) at Back (\"\")"="Data: Cleanup\nExit") -> ("States Out"=w726:string)  [unwired: 13 in]
        n304 = call <vilib>:"Add State(s) to Queue__JKI_lib_State_Machine.vi"("State(s) in Front (\"\")"=w726, "State(s) in (\"\")"=w735) -> ("States Out"=w734:string)  [unwired: 13 in]
      }
      frame "---------- New Category ----------" {
        # "Template Separator\n(You can make a copy of, or modify, this frame)"
        n305 = call <vilib>:"Add State(s) to Queue__JKI_lib_State_Machine.vi"("State(s) in (\"\")"=w740) -> ("States Out"=w739:string)  [unwired: 14 in]
      }
      frame "New Category: 1" {
        # "Your code here.\n(You can make a copy of, or modify, this frame)"
        n306 = call <vilib>:"Add State(s) to Queue__JKI_lib_State_Machine.vi"("State(s) in (\"\")"=w745) -> ("States Out"=w744:string)  [unwired: 14 in]
      }
      frame "New Category: 2" {
        # "Your code here.\n(You can make a copy of, or modify, this frame)"
        n307 = call <vilib>:"Add State(s) to Queue__JKI_lib_State_Machine.vi"("State(s) in (\"\")"=w750) -> ("States Out"=w749:string)  [unwired: 14 in]
      }
    }
  }
